vi "NextDown.vi"   [LabVIEW 2019, in "FloatUtil.lvlib"]
uses:
  FloatUtil.lvlib
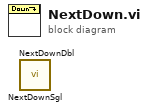
[diagram p0: block diagram]
diagram:
  n1 = call "NextDownSgl.vi"() -> ()  [unwired: 11 in, 1 out]
  n2 = call "NextDownDbl.vi"() -> ()  [unwired: 11 in, 1 out]
